vi "RawAttrMap.vi"() -> (3 "AttrMap":T1)   [LabVIEW 2019, in "lv-apt-json-file.lvlib"]
uses:
  lv-apt-json-file.lvlib
  Typedef/Def-AttrMap.ctl
  Typedef/Def-AttrMap -- Map.ctl
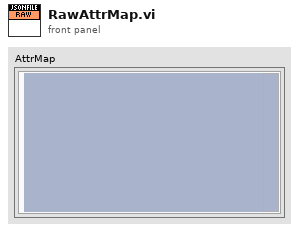
[diagram p1: front panel]
types:
  T1 = typedef "lv-apt-json-file.lvlib/Def-AttrMap.ctl" = cluster{"Map":variant}
  T2 = typedef "lv-apt-json-file.lvlib/Def-AttrMap -- Map.ctl" = map{string, string}
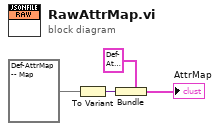
[diagram p0: block diagram]
diagram:
  n1 = To Variant(anything=T2 {}) -> (Variant=w4:variant)
  n2 = Bundle(cluster=T1 {"Map"=variant} ("AttrMap"), "Map"=w4) -> (→"AttrMap":T1)
